vi "Proxy_Extractvalues.vi"(11 "Read string":string) -> (0 "Header":string, 2 "Data - O2":dbl, 3 "Data - P":i16[](array[numeric]))   [LabVIEW 2019]
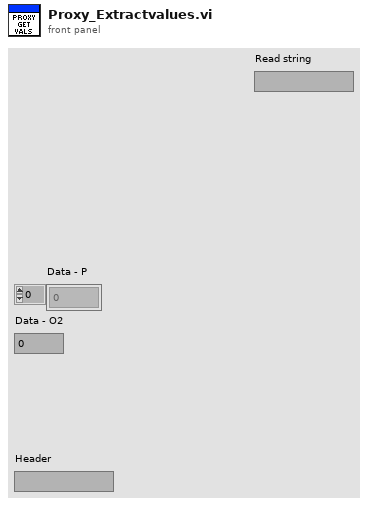
[diagram p1: front panel]
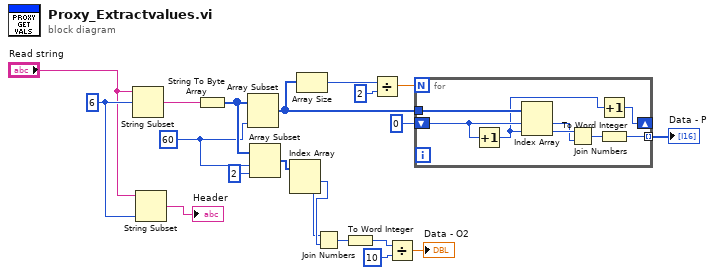
[diagram p0: block diagram]
diagram:
  w7 = 60 ("length")
  w20 = 6 ("length (rest)")
  n1 = String Subset(string="Read string", offset (0)=w20) -> (substring=w19:string)  [unwired: 1 in]
  n2 = String Subset(string="Read string", length (rest)=w20) -> (substring=→"Header":string)  [unwired: 1 in]
  n3 = String To Byte Array(string=w19) -> (unsigned byte array=w8:u8[])
  n4 = Array Subset(array=w8, length=w7) -> (w18:u8[])  [unwired: 1 in]
  n5 = Array Subset(array=w8, index=w7, length=2) -> (w4:u8[])
  n6 = Index Array(array=w4) -> (element #1=w3:u8, element #2=w2:u8)  [unwired: 2 in]
  n7 = Array Size(array=w18) -> (size(s)=w16:i32)
  n8 = Join Numbers(hi=w2, lo=w3) -> ((hi.lo)=w5:u16)
  n9 = To Word Integer(number=w5) -> (16bit integer=w1:i16)
  n10 = Divide(x=w16, y=2) -> (x/y=w15:dbl)
  n11 = Divide(x=w1, y=10) -> (x/y=→"Data - O2":dbl)
  n12 = for {
    N: w15 -> [_]
    tunnel: w18 -> [w28]
    shift-right: [w25] -> _
    shift-left: 0 ("y") -> [w27]
    tunnel: [w23] -> w14 mode=indexing
    n13 = Increment(x=w27) -> (x+1=w26:i32)
    n14 = Index Array(array=w28, index #1=w27, index #2=w26) -> (element #1=w21:u8, element #2=w22:u8)
    n15 = Join Numbers(hi=w22, lo=w21) -> ((hi.lo)=w24:u16)
    n16 = Increment(x=w26) -> (x+1=w25:i32)
    n17 = To Word Integer(number=w24) -> (16bit integer=w23:i16)
  }
  "Data - P" <- w14
